vi "log_goalie_scout.vi"() -> ()   [LabVIEW 2019]
panel:
  out "Velocity Graph":cluster{"X":dbl, "Y":dbl}[](graph)
  out "output string":string
  out "line index":i32=54857
  in  "stop":bool
  in  "file path (use dialog)":path=path "C:/AGV/Log/11/20201120551_md/Scout_1120551.txt"
  # "Scout log check"
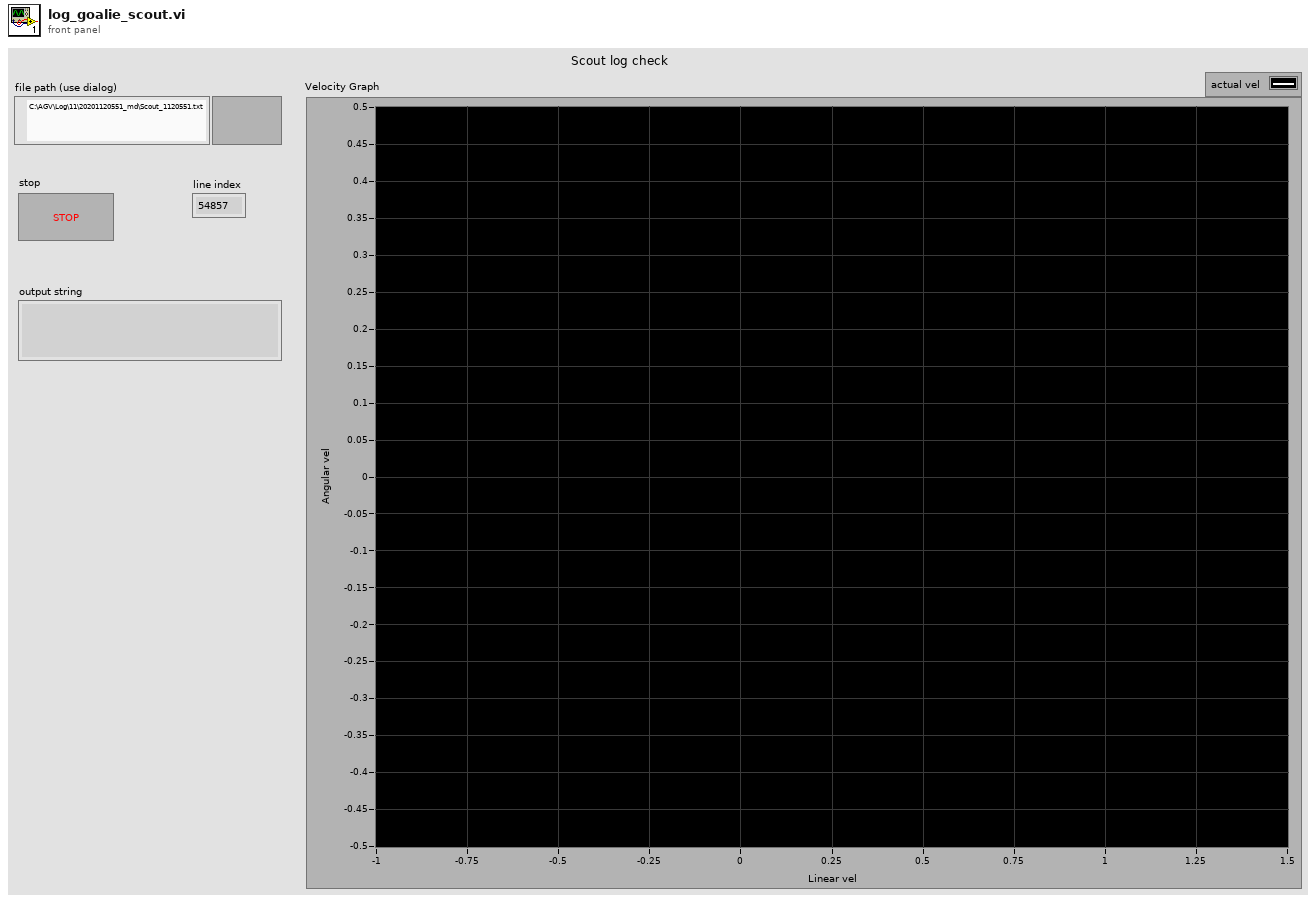
[diagram p1: front panel]
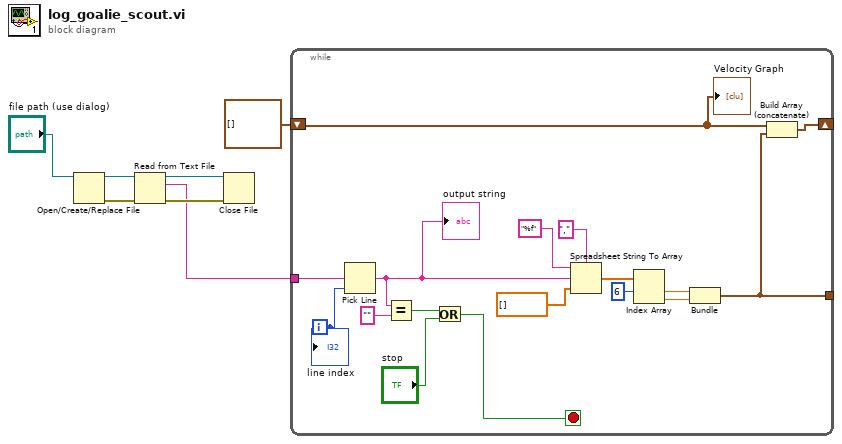
[diagram p0: block diagram]
diagram:
  n1 = Open/Create/Replace File(file path (use dialog)="file path (use dialog)") -> (refnum out=w7:refnum<file>, error out=w4:errorcluster)  [unwired: 5 in, 1 out]
  n2 = Read from Text File(file (use dialog)=w7, error in=w4) -> (refnum out=w6:refnum<file>, text=w2:string, error out=w5:errorcluster)  [unwired: 2 in, 1 out]
  n3 = Close File(refnum=w6, error in=w5) -> ()  [unwired: 2 out]
  n4 = while {
    tunnel: w2 -> [w24]
    tunnel: [w9] -> _
    shift-right: [w10] -> _
    shift-left: cluster{dbl, dbl}[] [] -> [w8]
    i -> [w23]
    stop <- w19 stop-if-true
    n5 = Pick Line(multi-line string=w24, line index=w23) -> (output string=w14:string)  [unwired: 1 in]
    "output string" <- w14
    n6 = Equal?(x=w14, y="") -> (x = y?=w21:bool)
    n7 = Or(x=w21, y="stop") -> (x .or. y?=w19:bool)
    n8 = Spreadsheet String To Array(delimiter (Tab)=",", format string="%f", spreadsheet string=w14, array type (2D Dbl)=dbl[] []) -> (array=w18:dbl[])
    n9 = Index Array(array=w18, index #1=6 ("index")) -> (element #1=w12:dbl, element #2=w11:dbl)  [unwired: 1 in]
    n10 = Bundle(w12, w11) -> (w9:cluster{dbl, dbl})  [unwired: 1 in]
    n11 = Build Array (concatenate)(w8, w9) -> (w10:cluster{dbl, dbl}[])
    "line index" <- w23
    "Velocity Graph" <- w8
  }
